vi "IMU2JointAngles2.vi"(6 "Operation(GetData)":T1, 7 "JointAngleDir (-1, 1, 1,-1)":dbl[](array[numeric])=[-1.0, 1.0, 1.0, -1.0], 8 "error in (no error)":errorcluster, 9 "LockHipAbduction(F)":bool, 10 "LockHipRotation(T)":bool=TRUE, 11 "IMU in (rad)":dbl[][](array[numeric])) -> (0 "error out":errorcluster, 3 "Joint Angles (rad)":dbl[](array[numeric]))   [LabVIEW 2016]
uses:
  TypeDef/IMU_operation.ctl
  <vilib>/Analysis/coordinate.llb/Euler Rotation Order.ctl
  <vilib>/Analysis/NI_AALPro.lvlib
panel:
  in  "UseStandPos(T)":bool=TRUE
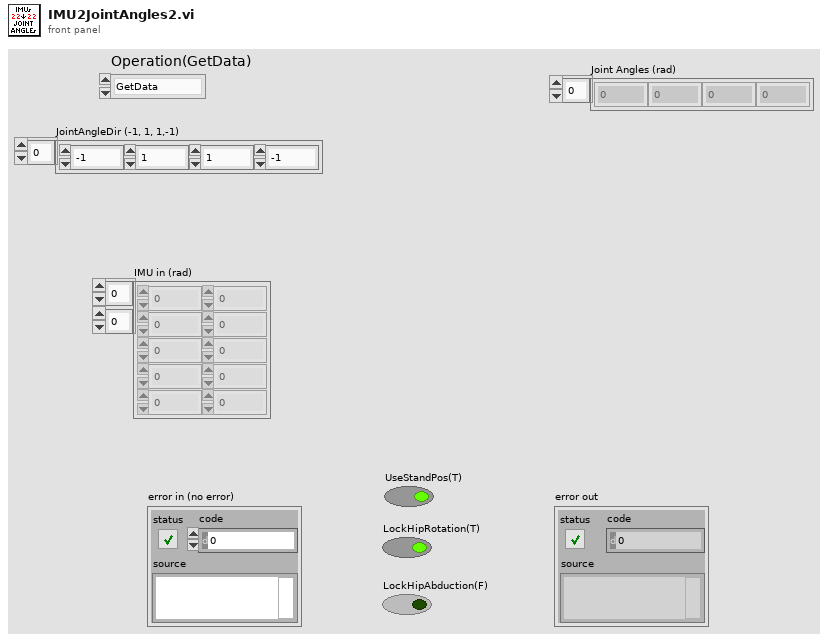
[diagram p1: front panel]
types:
  T1 = typedef "IMU_operation.ctl" = enum16{"GetData", "ClearStandPos", "SetStandPos"}
  T2 = typedef "NI_AALPro.lvlib/Euler Rotation Order.ctl" = u16
  T3 = cluster{"IMU in (rad)[0]":dbl, "IMU in (rad)[1]":dbl, "IMU in (rad)[2]":dbl}
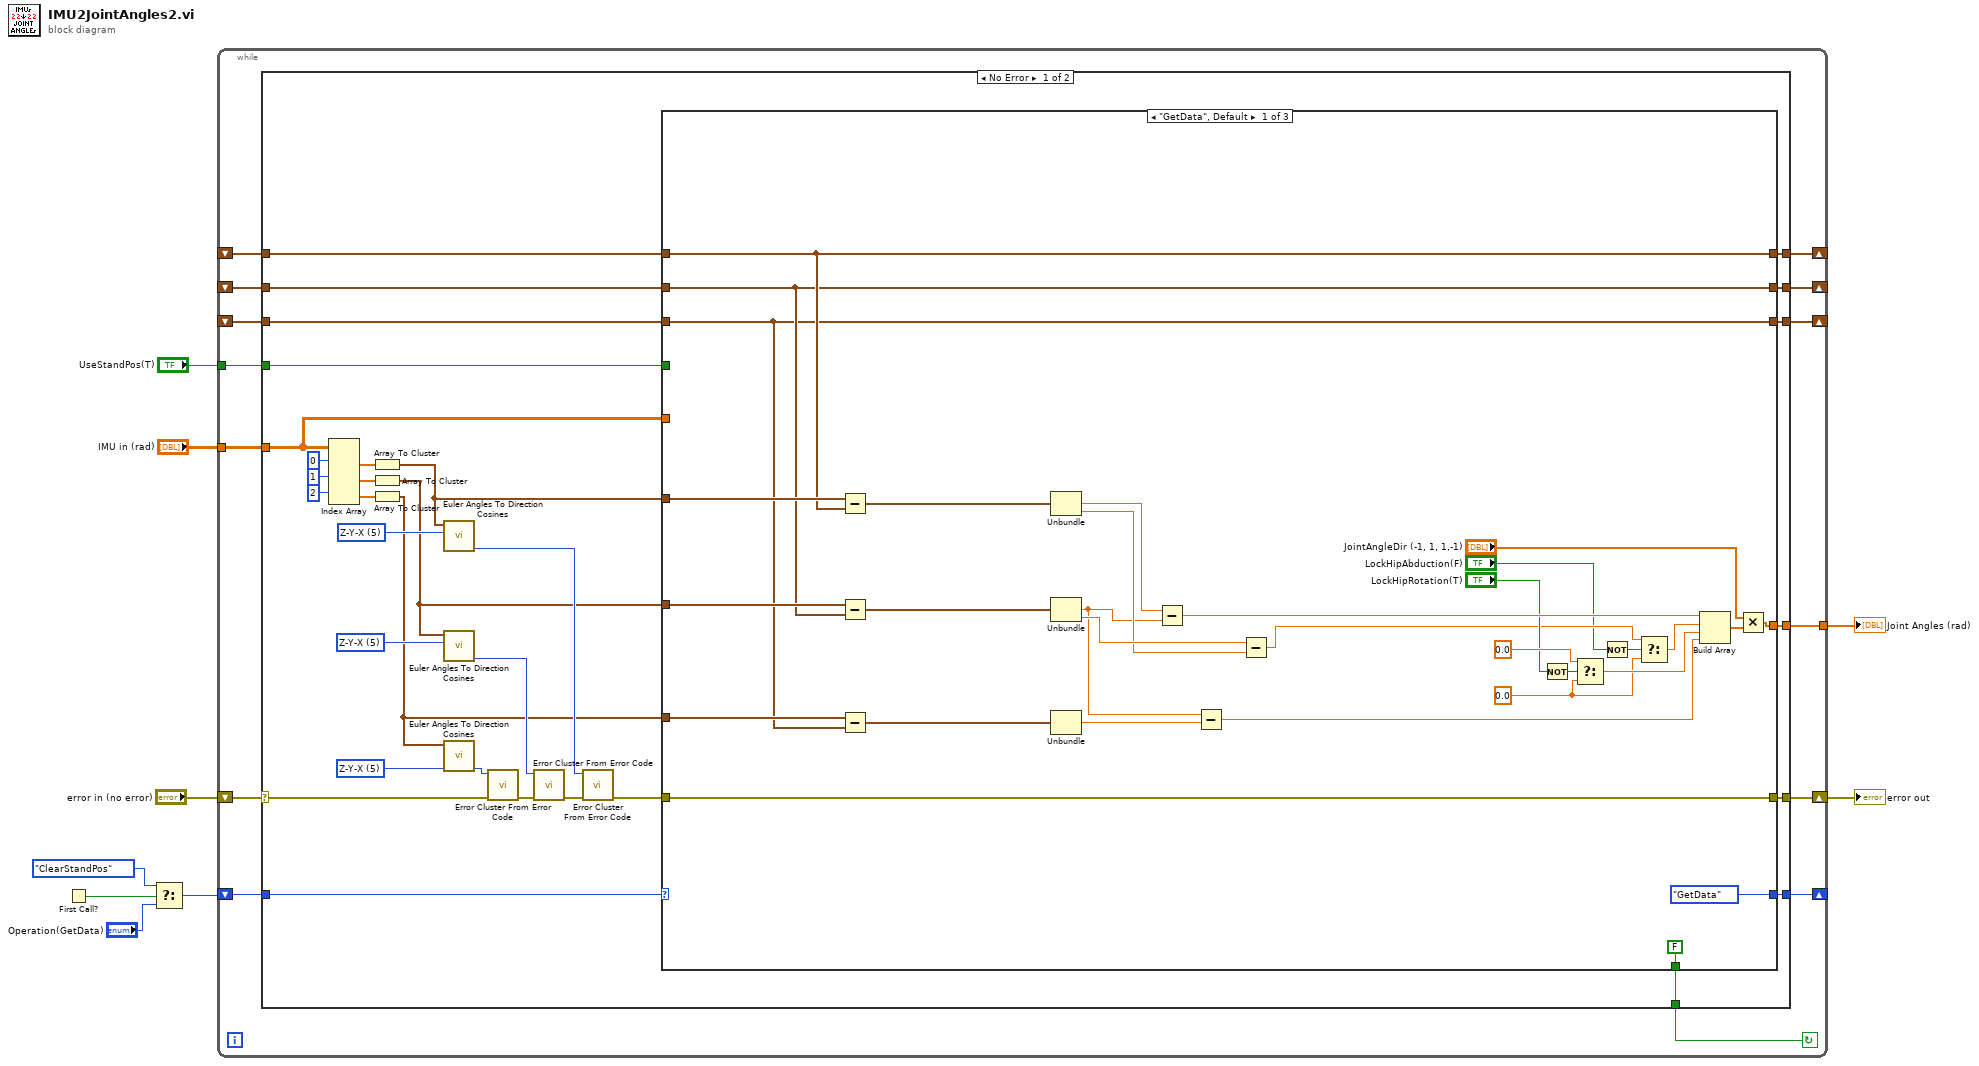
[diagram p0: block diagram]
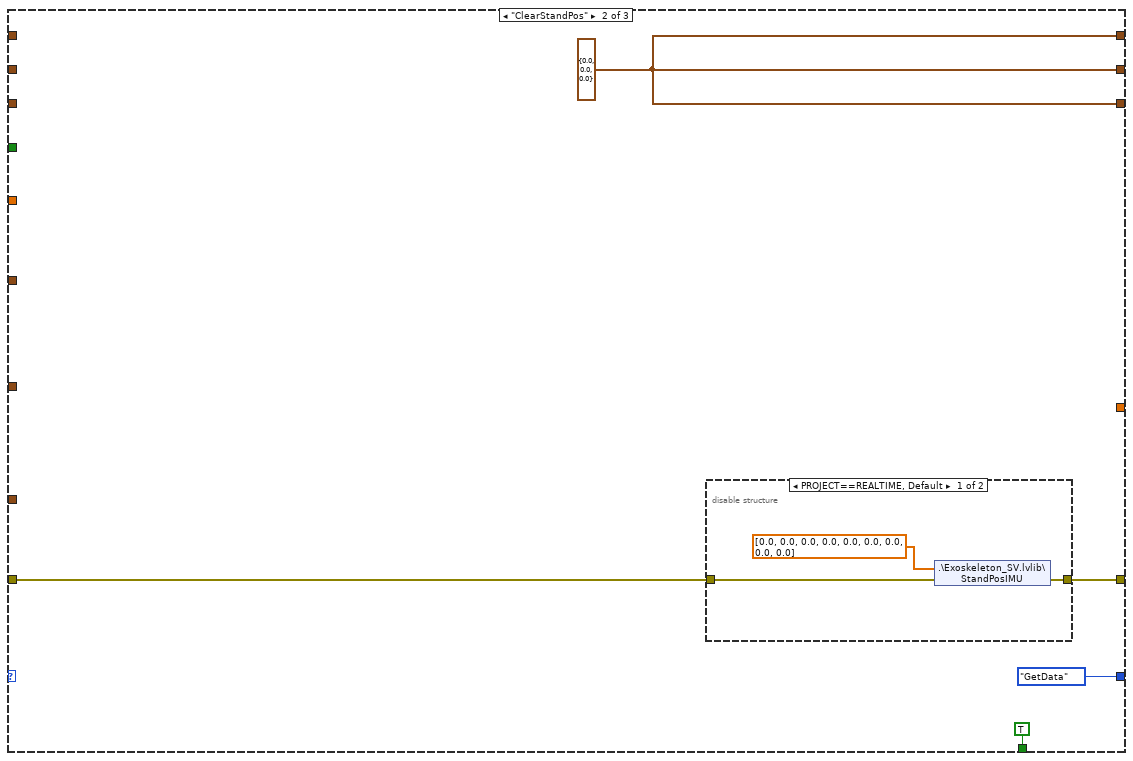
[diagram p2: hidden frame]
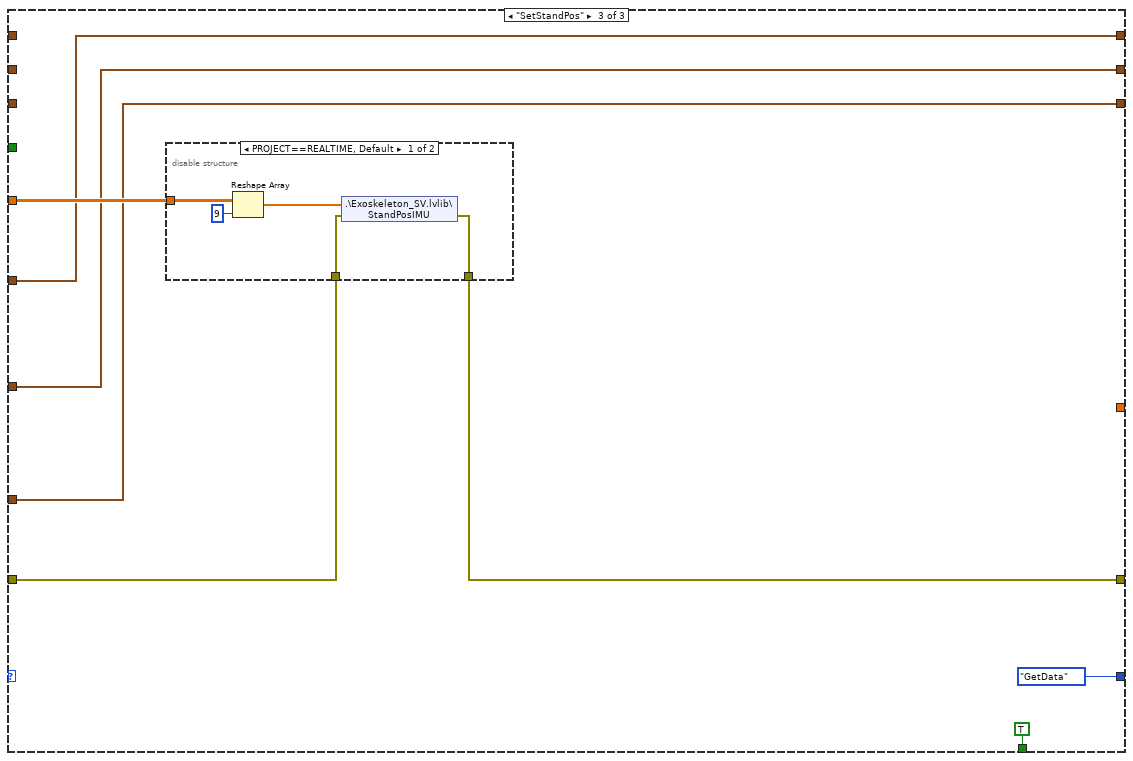
[diagram p4: hidden frame]
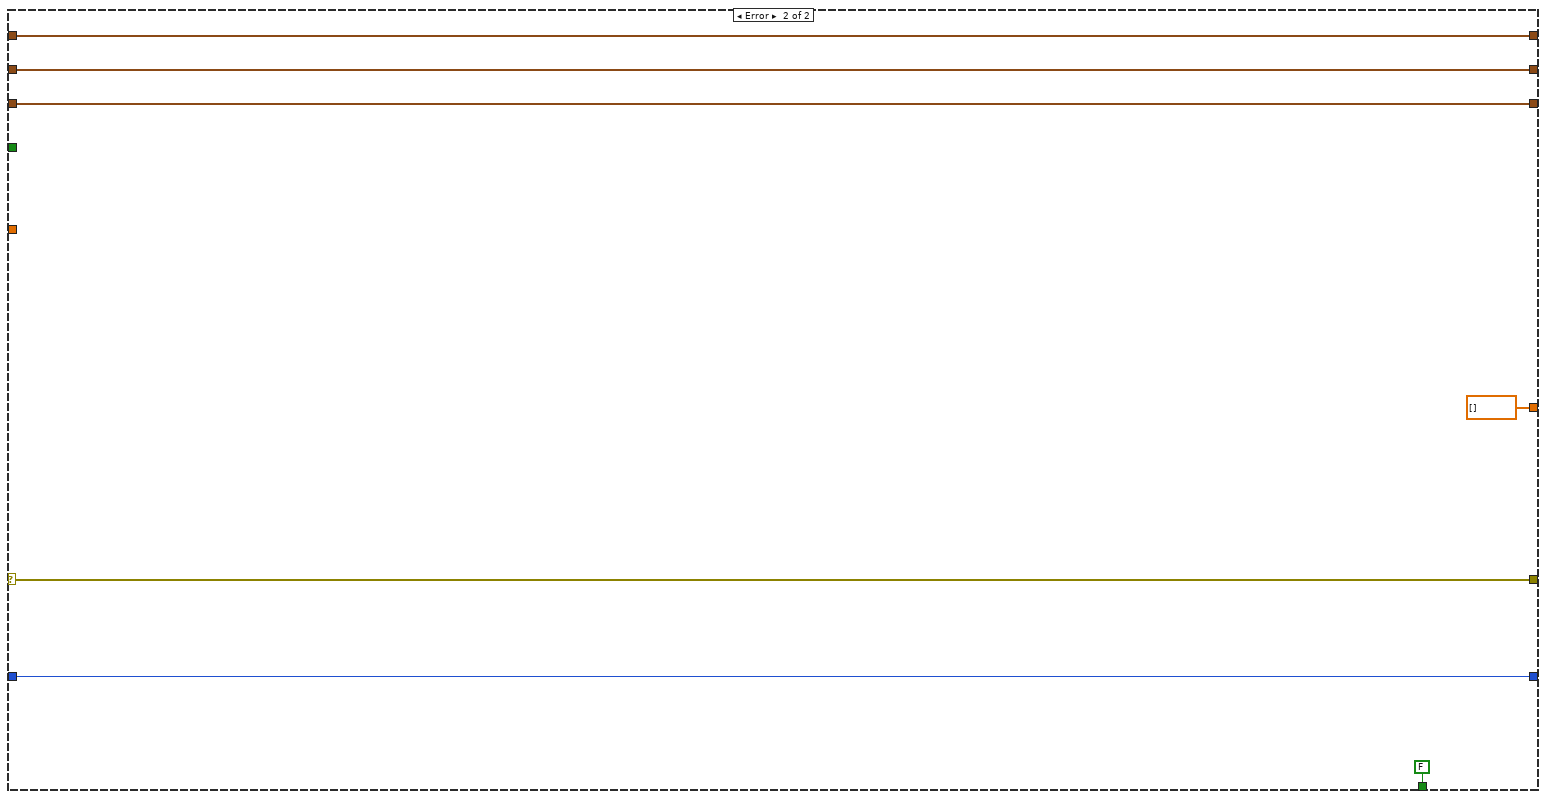
[diagram p6: hidden frame]
diagram:
  n1 = First Call?() -> (First Call?: T/F=w4:bool)
  n2 = Select(t=IMU_operation."ClearStandPos", s=w4, f="Operation(GetData)") -> (s? t:f=w2:T1)
  n3 = while {
    tunnel: [w23] -> w9
    tunnel: "IMU in (rad)" -> [w21]
    shift-right: [w20] -> w5
    shift-left: "error in (no error)" -> [w22]
    shift-right: [w10] -> _
    shift-left: w2 -> [w19]
    shift-right: [w18] -> _
    shift-left: _ -> [w14]
    shift-right: [w17] -> _
    shift-left: _ -> [w13]
    shift-right: [w16] -> _
    shift-left: _ -> [w12]
    tunnel: "UseStandPos(T)" -> [w11]
    stop <- w15 continue-if-true
    n4 = case shown="No Error" w22 {
      selector: w22 -> [w28 w112]
      tunnel: [w55 dbl[] []] -> w23
      tunnel: w21 -> [w27 _]
      tunnel: [w54 w112] -> w20
      tunnel: w19 -> [w53 w111]
      tunnel: [w52 w116] -> w18
      tunnel: [w51 w115] -> w17
      tunnel: [w50 w114] -> w16
      tunnel: [w49 FALSE] -> w15
      tunnel: w14 -> [w48 w116]
      tunnel: w13 -> [w47 w115]
      tunnel: w12 -> [w46 w114]
      tunnel: w11 -> [w45 _]
      tunnel: [w44 w111] -> w10
      frame No Error {
        w35 = T2 5 items=["X-Y-Z", "X-Z-Y", "Y-X-Z", "Y-Z-X", "Z-X-Y", "Z-Y-X", "X-Y-X", "X-Z-X", "Y-X-Y", "Y-Z-Y", "Z-X-Z", "Z-Y-Z"] ("rotation order")
        w36 = T2 5 items=["X-Y-Z", "X-Z-Y", "Y-X-Z", "Y-Z-X", "Z-X-Y", "Z-Y-X", "X-Y-X", "X-Z-X", "Y-X-Y", "Y-Z-Y", "Z-X-Z", "Z-Y-Z"] ("rotation order")
        w37 = T2 5 items=["X-Y-Z", "X-Z-Y", "Y-X-Z", "Y-Z-X", "Z-X-Y", "Z-Y-X", "X-Y-X", "X-Z-X", "Y-X-Y", "Y-Z-Y", "Z-X-Z", "Z-Y-Z"] ("rotation order")
        n5 = Index Array(array=w27, index (row) #1=0 ("index (row)"), index (row) #2=1 ("index (row)"), index (row) #3=2 ("index (row)")) -> (element #1=w38:dbl[], element #2=w40:dbl[], element #3=w39:dbl[])  [unwired: 3 in]
        n6 = Array To Cluster(array=w38) -> (cluster=w24:T3)
        n7 = Array To Cluster(array=w40) -> (cluster=w25:T3)
        n8 = Array To Cluster(array=w39) -> (cluster=w26:T3)
        n9 = call <vilib>:"Euler Angles To Direction Cosines.vi"("rotation order"=w35, "Euler Angles"=w24) -> ("error"=w34:i32)  [unwired: 8 in, 1 out]
        n10 = call <vilib>:"Euler Angles To Direction Cosines.vi"("rotation order"=w37, "Euler Angles"=w25) -> ("error"=w33:i32)  [unwired: 8 in, 1 out]
        n11 = call <vilib>:"Euler Angles To Direction Cosines.vi"("rotation order"=w36, "Euler Angles"=w26) -> ("error"=w32:i32)  [unwired: 8 in, 1 out]
        n12 = call <vilib>:"Error Cluster From Error Code.vi"("error in (no error)"=w28, "error code (0)"=w32) -> ("error out"=w31:errorcluster)  [unwired: 7 in]
        n13 = call <vilib>:"Error Cluster From Error Code.vi"("error in (no error)"=w31, "error code (0)"=w33) -> ("error out"=w30:errorcluster)  [unwired: 7 in]
        n14 = call <vilib>:"Error Cluster From Error Code.vi"("error in (no error)"=w30, "error code (0)"=w34) -> ("error out"=w29:errorcluster)  [unwired: 7 in]
        n15 = case shown="\"GetData\", Default" w53 {
          tunnel: [w85 _ _] -> w55
          tunnel: w29 -> [w78 w88 w102]
          tunnel: w27 -> [_ _ w103]
          tunnel: [w78 w91 w99] -> w54
          tunnel: [w66 w87 w97] -> w52
          tunnel: [w62 w87 w98] -> w51
          tunnel: [w59 w87 w96] -> w50
          tunnel: [FALSE TRUE TRUE] -> w49
          tunnel: w48 -> [w66 _ _]
          tunnel: w47 -> [w62 _ _]
          tunnel: w46 -> [w59 _ _]
          tunnel: w45 -> [_ _ _]
          tunnel: [IMU_operation."GetData" ("Operation(GetData)") IMU_operation."GetData" ("Operation(GetData)") IMU_operation."GetData" ("Operation(GetData)")] -> w44
          tunnel: w26 -> [w61 _ w96]
          tunnel: w25 -> [w64 _ w98]
          tunnel: w24 -> [w67 _ w97]
          frame "GetData", Default {
            w71 = 0.0 ("psi")
            n16 = Subtract(x=w67, y=w66) -> (x-y=w65:T3)
            n17 = Subtract(x=w64, y=w62) -> (x-y=w63:T3)
            n18 = Subtract(x=w61, y=w59) -> (x-y=w60:T3)
            n19 = Unbundle(w65) -> ("IMU in (rad)[1]"=w58:dbl, "IMU in (rad)[2]"=w68:dbl)  [unwired: 1 out]
            n20 = Unbundle(w63) -> ("IMU in (rad)[1]"=w56:dbl, "IMU in (rad)[2]"=w69:dbl)  [unwired: 1 out]
            n21 = Unbundle(w60) -> ("IMU in (rad)[1]"=w57:dbl)  [unwired: 2 out]
            n22 = Subtract(x=w58, y=w56) -> (x-y=w83:dbl)
            n23 = Subtract(x=w56, y=w57) -> (x-y=w82:dbl)
            n24 = Subtract(x=w69, y=w68) -> (x-y=w73:dbl)
            n25 = Not(x="LockHipRotation(T)") -> (.not. x?=w74:bool)
            n26 = Select(t=0.0 ("psi"), s=w74, f=w71) -> (s? t:f=w76:dbl)
            n27 = Not(x="LockHipAbduction(F)") -> (.not. x?=w70:bool)
            n28 = Select(t=w73, s=w70, f=w71) -> (s? t:f=w81:dbl)
            n29 = Build Array(w83, w81, w76, w82) -> (w86:dbl[])
            n30 = Multiply(x="JointAngleDir (-1, 1, 1,-1)", y=w86) -> (x*y=w85:dbl[])
          }
          frame "ClearStandPos" {
            w87 = T3 {"IMU in (rad)[0]"=0.0, "IMU in (rad)[1]"=0.0, "IMU in (rad)[2]"=0.0} ("IMU in (rad)")
            n31 = disable-structure shown="PROJECT==REALTIME, Default" {
              disable-tunnel: w88 -> [w93 w95]
              disable-tunnel: [w92 w95] -> w91
              frame condition #0 (active) {
                n32 = shared-variable ".\\Exoskeleton_SV.lvlib\\StandPosIMU"(dbl[] [0.0, 0.0, 0.0, 0.0, 0.0, 0.0, 0.0, 0.0, 0.0] ("ZeroOrient"), error in=w93) -> (error out=w92:errorcluster)
              }
              frame condition #1 {
              }
            }
          }
          frame "SetStandPos" {
            n33 = disable-structure shown="PROJECT==REALTIME, Default" {
              disable-tunnel: w103 -> [w107 _]
              disable-tunnel: w102 -> [w105 w109]
              disable-tunnel: [w104 w109] -> w99
              frame condition #0 (active) {
                n34 = Reshape Array(w107, 9 ("dimension size")) -> (w106:dbl[])
                n35 = shared-variable ".\\Exoskeleton_SV.lvlib\\StandPosIMU"(w106, error in=w105) -> (error out=w104:errorcluster)
              }
              frame condition #1 {
              }
            }
          }
        }
      }
      frame Error {
      }
    }
  }
  "Joint Angles (rad)" <- w9
  "error out" <- w5
